vi "Stop SubActors.vi"(11 "SuperActor in":refnum<class "SuperActor.lvclass">) -> (3 "SuperActor out":refnum<class "SuperActor.lvclass">)   [LabVIEW 2016, in "SuperActor.lvlib" / "SuperActor.lvclass"]
uses:
  SuperActor.lvclass
  C:/Program Files (x86)/National Instruments/LabVIEW 2016/vi.lib/ActorFramework/Actor/Actor.lvclass
  SuperActor.lvclass/SuperActor.ctl
  <vilib>/ActorFramework/Actor/Actor.lvclass/Actor.ctl
  <vilib>/ActorFramework/Message Enqueuer/Message Enqueuer.lvclass/Message Enqueuer.ctl
  <vilib>/ActorFramework/Message Enqueuer/Message Enqueuer.lvclass
  <vilib>/ActorFramework/Message Enqueuer/Init from Existing Queue.vi
  <vilib>/ActorFramework/Message Enqueuer/Enqueue.vi
  <vilib>/ActorFramework/Stop Msg/Stop Msg.lvclass
  C:/Program Files (x86)/National Instruments/LabVIEW 2016/vi.lib/ActorFramework/Message/Message.lvclass
  <vilib>/ActorFramework/Message Priority Queue/Priority Enqueue.vi
  Session APIs/Session Log/System Log.lvclass
  <vilib>/ActorFramework/Actor/Actor.lvclass
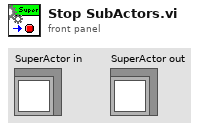
[diagram p1: front panel]
types:
  T1 = typedef "Session - Root.lvclass/Session Handle.ctl" = refnum<data-value>
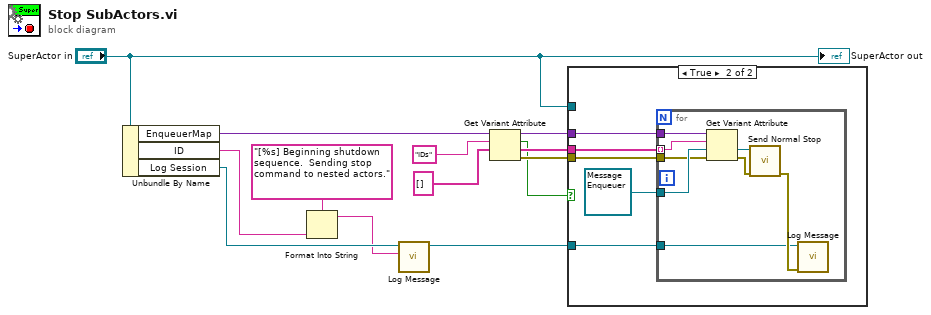
[diagram p0: block diagram]
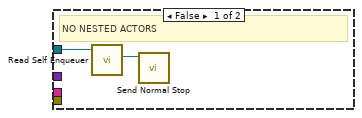
[diagram p2: hidden frame]
diagram:
  n1 = Unbundle By Name("SuperActor in") -> ("EnqueuerMap"=w13:variant, "ID"=w7:string, "Log Session"=w8:T1)
  n2 = Format Into String(format string="[%s] Beginning shutdown sequence.  Sending stop command to nested actors.", w7) -> (resulting string=w5:string)  [unwired: 2 in, 1 out]
  n3 = call "Log Message.vi"("MSG In"=w5, "session in"=w8) -> ("session out"=w3:T1)  [unwired: 8 in, 1 out]
  n4 = Get Variant Attribute(Variant=w13, name="IDs", default value (empty Variant)=string[] []) -> (duplicate Variant=w9:variant, found=w2:bool, value=w10:string[], error out=w4:errorcluster)  [unwired: 1 in]
  n5 = case shown="True" w2 {
    tunnel: w10 -> [_ w20]
    tunnel: w9 -> [_ w19]
    tunnel: w4 -> [_ w17]
    tunnel: w3 -> [_ w16]
    tunnel: "SuperActor in" -> [w15 _]
    frame False {
      # "NO NESTED ACTORS"
      n6 = call <vilib>:"Read Self Enqueuer.vi"("Actor"=w15) -> ("Self Enqueuer"=w14:refnum<class "Message Enqueuer.lvclass">)  [unwired: 10 in]
      n7 = call <vilib>:"Send Normal Stop.vi"("Message Enqueuer"=w14) -> ()  [unwired: 10 in, 1 out]
    }
    frame True {
      n8 = for {
        tunnel: w20 -> [w27] mode=indexing
        tunnel: w19 -> [w28]
        tunnel: refnum<class "Message Enqueuer.lvclass"> refnum ("Message Enqueuer in") -> [w26]
        tunnel: w17 -> [w24]
        tunnel: w16 -> [w21]
        n9 = Get Variant Attribute(Variant=w28, name=w27, default value (empty Variant)=w26, error in=w24) -> (value=w25:refnum<class "Message Enqueuer.lvclass">, error out=w23:errorcluster)  [unwired: 2 out]
        n10 = call <vilib>:"Send Normal Stop.vi"("error in (no error)"=w23, "Message Enqueuer"=w25) -> ("error out"=w22:errorcluster)  [unwired: 9 in]
        n11 = call "Log Message.vi"("error in"=w22, "session in"=w21) -> ()  [unwired: 8 in, 2 out]
      }
    }
  }
  "SuperActor out" <- "SuperActor in"
